vi "DC2100 Close.vi"(8 "error in (no error)":errorcluster, 11 "instrument handle":refnum<visa-resource-name>) -> (0 "error out":errorcluster)   [LabVIEW 2019]
doc: "This function closes the instrument driver session and the VISA Resource Manager session.\n\nNote: The instrument must be reinitialized to use it again."
uses:
  DC2100_Drv_32.dll
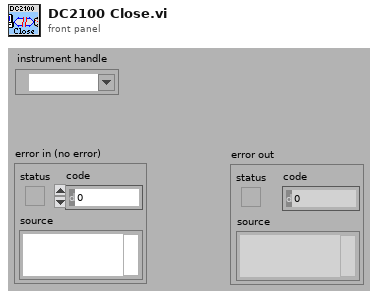
[diagram p1: front panel]
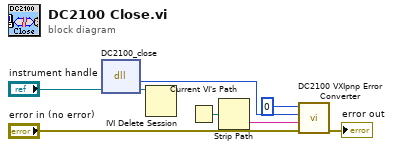
[diagram p0: block diagram]
diagram:
  n1 = dll-call lib="C:/Users/mdrohr/Documents/GitHub/cerebral-hemodynamics/blood-oxygenation/DC2100_Drv_32.dll" fn="DC2100_close"("instrument handle"="instrument handle") -> ("status"=w4:i32)  [unwired: 4 in, 2 out]
  n2 = IVI Delete Session(11:"instrument handle") -> ()
  n3 = Current VI's Path() -> (path=w7:path)
  n4 = Strip Path(path=w7) -> (name=w3:string)  [unwired: 1 out]
  n5 = call "DC2100 VXIpnp Error Converter.vi"("error in (no error)"="error in (no error)", "name of VI (\"\")"=w3, "CVI error code (0)"=w4, "instrument handle"=i8 0) -> ("error out"=→"error out":errorcluster)  [unwired: 6 in, 1 out]
